vi "Generador_De_Pistas.vi"(1 "Num_Columnas":dbl, 2 "Num_Filas":dbl, 3 "Posiciones_Minas":string[](array[string])) -> (0 "Pistas":T1(array[cluster]))   [LabVIEW 2019]
doc: "Parametros: -----------------------------------------\n\n'Posiciones_Minas': lista con cadenas 'x,y' donde x e y corresponden a la posicion de la mina en el tablero.\n\n'Num_Filas': corresponde al número total de filas que contiene el tablero.\n\n'Num_Columnas': corresponde al número total de columnas que contiene el tablero.tablero.\n\nRetorna: -------------------------------------------------------\n\n'Pistas': Lista de clusteres conformados por un String 'x,y' correspondiente a la posicion de la pista y un entero que indica el numero de minas alrededor de la pista."
uses:
  70c9b82d-3797-480a-9f21-1e4d1ee8be6b.vi
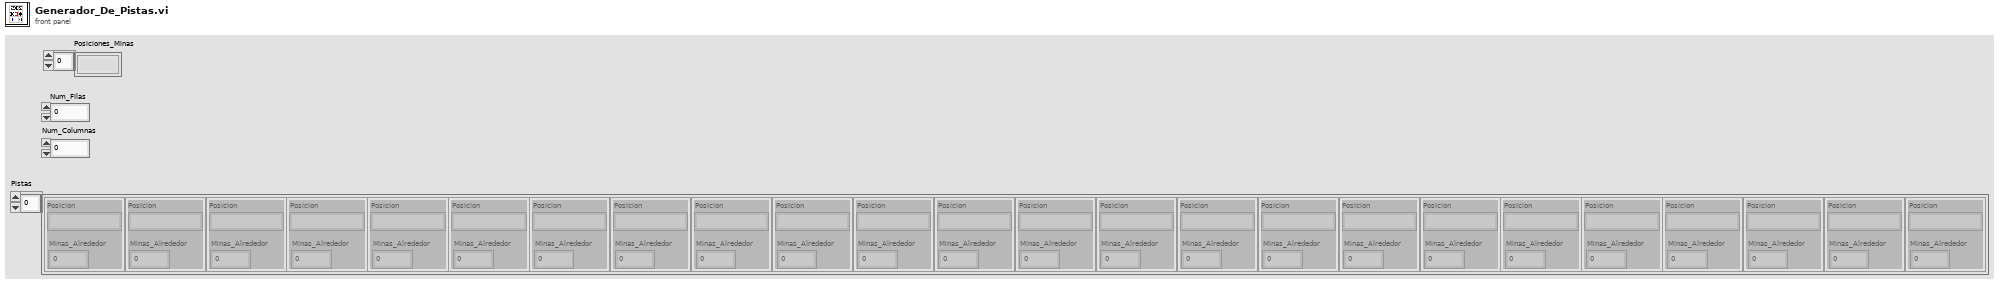
[diagram p1: front panel]
types:
  T1 = cluster{"Posicion":string, "Minas_Alrededor":dbl}[]
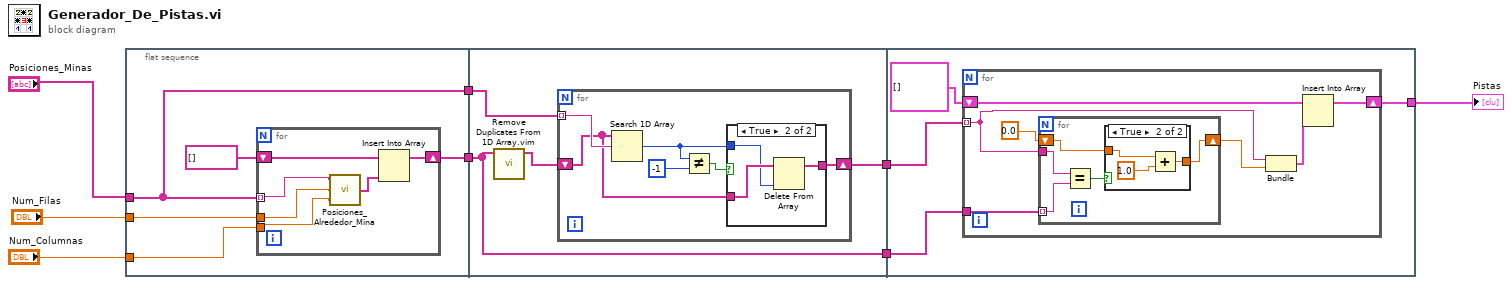
[diagram p0: block diagram]
diagram:
  n1 = flat-sequence {
    tunnel: "Posiciones_Minas" -> [w10]
    tunnel: "Num_Filas" -> [w13]
    tunnel: [w11] -> w8
    tunnel: [w10] -> w7
    tunnel: "Num_Columnas" -> [w9]
    tunnel: w8 -> [w20]
    tunnel: w7 -> [w23]
    tunnel: [w21] -> w6
    tunnel: [w20] -> w5
    tunnel: w6 -> [w37]
    tunnel: w5 -> [w36]
    tunnel: [w34] -> w4
    frame #0 {
      n2 = for {
        tunnel: w10 -> [w17] mode=indexing
        tunnel: w13 -> [w16]
        shift-right: [w19] -> w11
        shift-left: string[] [] -> [w18]
        tunnel: w9 -> [w15]
        n3 = call "Posiciones_Alrededor_Mina.vi"("Numero_Columnas"=w15, "Numero_Filas"=w16, "Posicion"=w17) -> ("Posiciones_Alrededor_Mina"=w14:string[])
        n4 = Insert Into Array(array=w18, new element=w14) -> (w19:string[])  [unwired: 1 in]
      }
    }
    frame #1 {
      n5 = call "Remove Duplicates From 1D Array.vim"("array"=w20) -> ("array with duplicates removed"=w22:string[])  [unwired: 10 in]
      n6 = for {
        tunnel: w23 -> [w29] mode=indexing
        shift-right: [w25] -> w21
        shift-left: w22 -> [w28]
        n7 = Search 1D Array(1D array=w28, element=w29) -> (index of element=w24:i32)  [unwired: 1 in]
        n8 = Not Equal?(x=w24, y=-1) -> (x != y?=w26:bool)
        n9 = case shown="True" w26 {
          tunnel: w28 -> [w30 w33]
          tunnel: w24 -> [_ w32]
          tunnel: [w30 w31] -> w25
          frame False {
          }
          frame True {
            n10 = Delete From Array(array=w33, index=w32) -> (array with subset deleted=w31:string[])  [unwired: 1 in, 1 out]
          }
        }
      }
    }
    frame #2 {
      n11 = for {
        tunnel: w37 -> [w41] mode=indexing
        tunnel: w36 -> [w44]
        shift-right: [w39] -> w34
        shift-left: cluster{"Posicion_Inferior":string, dbl}[] [] -> [w38]
        n12 = for {
          tunnel: w44 -> [w48] mode=indexing
          tunnel: w41 -> [w49]
          shift-right: [w46] -> w42
          shift-left: 0.0 -> [w45]
          n13 = Equal?(x=w49, y=w48) -> (x = y?=w47:bool)
          n14 = case shown="True" w47 {
            tunnel: [w50 w52] -> w46
            tunnel: w45 -> [w50 w51]
            frame False {
            }
            frame True {
              n15 = Add(x=w51, y=1.0) -> (x+y=w52:dbl)
            }
          }
        }
        n16 = Bundle("Posicion_Inferior"=w41, w42) -> (w40:cluster{"Posicion_Inferior":string, dbl})  [unwired: 1 in]
        n17 = Insert Into Array(array=w38, new element=w40) -> (w39:cluster{"Posicion_Inferior":string, dbl}[])  [unwired: 1 in]
      }
    }
  }
  "Pistas" <- w4
